vi "tankdrive.vi"() -> ()   [LabVIEW 2012, in "Omni2013.lvrbt"]
uses:
  Omni2013.lvrbt
  <vilib>/NXT/Hardware/Plugins/Tetrix DC Motor/TetrixDCMotorAddress.ctl
  <vilib>/FTC/FTC Calculate Drive Power - Arcade Left.vi
  <vilib>/NXT/Dual Mode Library/Display/drawNumber.vi
  <vilib>/NXT/NXTIO Xnodes/NXTIONodeSubVIs/TETRIX IO Move DC Motors.vi
  <vilib>/NXT/Dual Mode Library/Display/drawText_Center.vi
  <vilib>/NXT/Subs/LVHSConnector.ctl
  <vilib>/NXT/NXTIO Xnodes/AddressXNode/NXTIOAddress.xnode
  <vilib>/NXT/NXTIO Xnodes/NXTIOXNode/NXTIO.xnode
  <vilib>/NXT/LegoClasses/BrickReference/BrickReference.lvclass
panel:
  in  "Drive Power":i8=100 min=-100 max=100
  # "This VI was generated based on your configuration in the Remote Control Editor. You may modify the code as needed for your robot. To test this program for an FTC match, return to the Remote Control Editor, select the \"Run Program\" tab, and choose \"FTC Game\"."
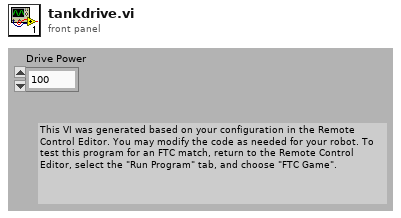
[diagram p1: front panel]
types:
  T1 = typedef "LVHSConnector.ctl" = refnum<class "BrickReference.lvclass">
  T2 = typedef "FTC ControllerState.ctl" = cluster{"Left X":i8, "Left Y":i8, "Right X":i8, "Right Y":i8, "Button Encoding 9-12":u8, "Button Encoding 1-8":u8, "POV":T3}
  T3 = typedef "FTC POVState.ctl" = i8
  T4 = typedef "TetrixDCMotorAddress.ctl" = i16
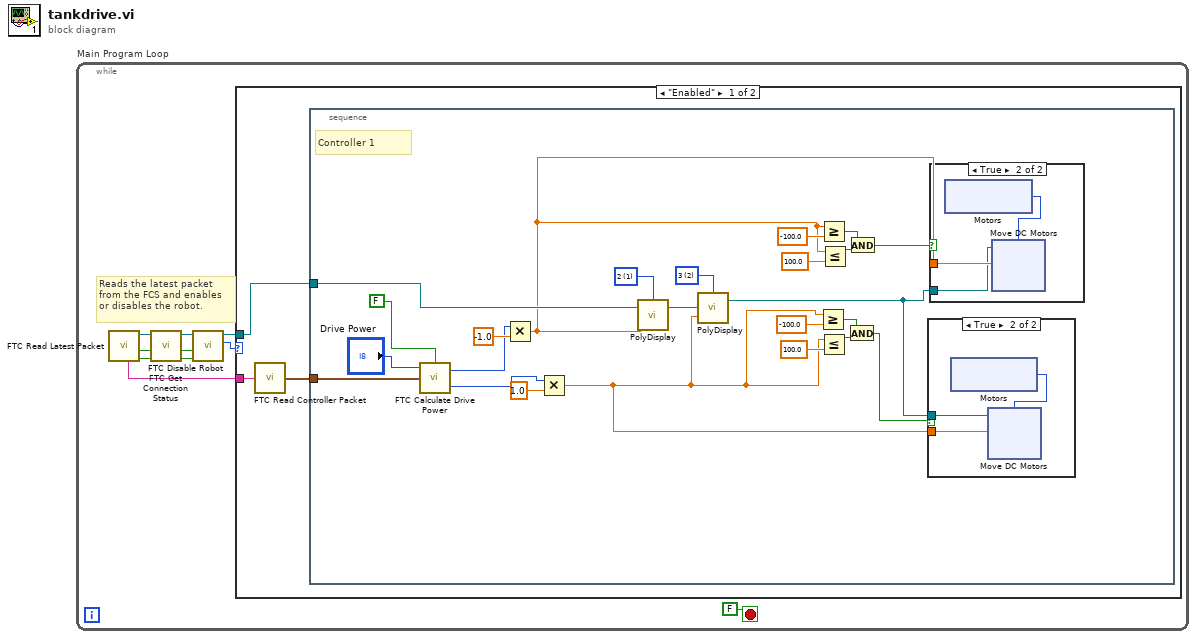
[diagram p0: block diagram]
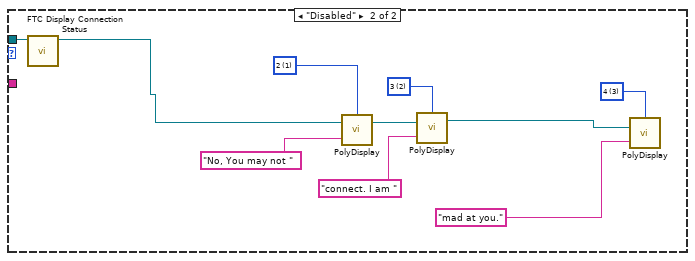
[diagram p4: hidden frame]
diagram:
  n1 = while "Main Program Loop" {
    stop <- FALSE stop-if-true
    # "Reads the latest packet\nfrom the FCS and enables\nor disables the robot."
    n2 = call <vilib>:"FTC Read Latest Packet.vi"() -> ("Packet Received?"=w8:bool, "Stopped?"=w5:bool, "NXT"=w7:T1, "Controller 1"=w9:string)  [unwired: 6 in, 2 out]
    n3 = call <vilib>:"FTC Get Connection Status.vi"("Packet Received?"=w8, "Stopped?"=w5, "NXT"=w7) -> ("Online?"=w2:bool, "Stopped?"=w3:bool, "NXT"=w4:T1)  [unwired: 5 in]
    n4 = call <vilib>:"FTC Disable Robot.vi"("Online?"=w2, "Stopped?"=w3, "NXT"=w4) -> ("Enabled?"=w6:enum16{"Disabled", "Enabled"}, "NXT"=w1:T1)  [unwired: 3 in]
    n5 = case "disableCase" shown="\"Enabled\"" w6 {
      tunnel: w9 -> [w13 _]
      tunnel: w1 -> [w11 w69]
      frame "Enabled" {
        n6 = call <vilib>:"FTC Read Controller Packet.vi"("Packet"=w13) -> ("Controller State"=w12:T2)  [unwired: 4 in]
        n7 = stacked-sequence "controller1Actions" {
          tunnel: w12 -> [w37]
          tunnel: w11 -> [w28]
          frame #0 {
            w33 = i16 2 items=["1", "2", "3", "4", "5", "6", "7", "8"] ("Line")
            w34 = i16 1 items=["1", "2", "3", "4", "5", "6", "7", "8"] ("Line")
            # "Controller 1"
            n8 = call-poly <vilib>:"FTC Calculate Drive Power.vi"("Reverse"=FALSE, "Controller State"=w37, "Power Level (50)"="Drive Power") -> ("Right Motor Power"=w29:i8, "Left Motor Power"=w30:i8)  [unwired: 1 in]
            n9 = Multiply(x=w30, y=-1.0) -> (x*y=w17:dbl)
            n10 = Multiply(x=w29, y=1.0) -> (x*y=w15:dbl)
            n11 = call-poly <vilib>:"PolyDisplay.vi"("number"=w17, "NXT"=w28, "Line"=w34) -> ("NXT"=w27:T1)  [unwired: 1 in]
            n12 = call-poly <vilib>:"PolyDisplay.vi"("number"=w15, "NXT"=w27, "Line"=w33) -> ("NXT"=w14:T1)  [unwired: 1 in]
            n13 = Greater Or Equal?(x=w15, y=-100.0) -> (x >= y?=w19:bool)
            n14 = Greater Or Equal?(x=w17, y=-100.0) -> (x >= y?=w23:bool)
            n15 = Less Or Equal?(x=w15, y=100.0) -> (x <= y?=w20:bool)
            n16 = Less Or Equal?(x=w17, y=100.0) -> (x <= y?=w24:bool)
            n17 = And(x=w19, y=w20) -> (x .and. y?=w16:bool)
            n18 = And(x=w23, y=w24) -> (x .and. y?=w18:bool)
            n19 = case shown="True" w16 {
              tunnel: w15 -> [_ w51]
              tunnel: w14 -> [_ w49]
              frame False {
              }
              frame True {
                n20 = xnode ("Motors")() -> ("Motor"=w50:T4)
                n21 = xnode ("Move DC Motors")("Power/Speed 1"=w51, "Motors"=w50, "NXT"=w49) -> ()  [unwired: 1 out]
              }
            }
            n22 = case shown="True" w18 {
              tunnel: w17 -> [_ w40]
              tunnel: w14 -> [_ w38]
              frame False {
              }
              frame True {
                n23 = xnode ("Motors")() -> ("Motor"=w39:T4)
                n24 = xnode ("Move DC Motors")("Power/Speed 1"=w40, "Motors"=w39, "NXT"=w38) -> ()  [unwired: 1 out]
              }
            }
          }
        }
      }
      frame "Disabled" {
        w63 = i16 3 items=["1", "2", "3", "4", "5", "6", "7", "8"] ("Line")
        w68 = i16 2 items=["1", "2", "3", "4", "5", "6", "7", "8"] ("Line")
        w64 = i16 1 items=["1", "2", "3", "4", "5", "6", "7", "8"] ("Line")
        n25 = call <vilib>:"FTC Display Connection Status.vi"("NXT"=w69) -> ("NXT"=w60:T1)  [unwired: 10 in]
        n26 = call-poly <vilib>:"PolyDisplay.vi"("Text"="No, You may not ", "NXT"=w60, "Line"=w64) -> ("NXT"=w66:T1)  [unwired: 1 in]
        n27 = call-poly <vilib>:"PolyDisplay.vi"("Text"="connect. I am ", "NXT"=w66, "Line"=w68) -> ("NXT"=w62:T1)  [unwired: 1 in]
        n28 = call-poly <vilib>:"PolyDisplay.vi"("Text"="mad at you.", "NXT"=w62, "Line"=w63) -> ()  [unwired: 1 in, 1 out]
      }
    }
  }
